vi "Core-ErrorHandler.vi"(7 "Ctrl-Refs":T1, 8 "Err-I":errorcluster, 9 "DaqQ-I":refnum<queue>, 10 "MainQ-I":refnum<queue>, 11 "ErrQ-I":refnum<queue>) -> (0 "Err-O":errorcluster)   [LabVIEW 2020]
doc: "CORE-ERROR HANDLING LOOP."
uses:
  Core-CtrlRefs.ctl
panel:
  # ":: Modularized Parallism Templete ::\n- Error Handling Loop -\nby: Techie <HighTechYoung@yahoo.com>\nhttp://www.Vigo-tech.com\nCopyright (C) 2010, Vigo Technologies All Rights Reserved"
  # "Outputs"
  # "Inputs"
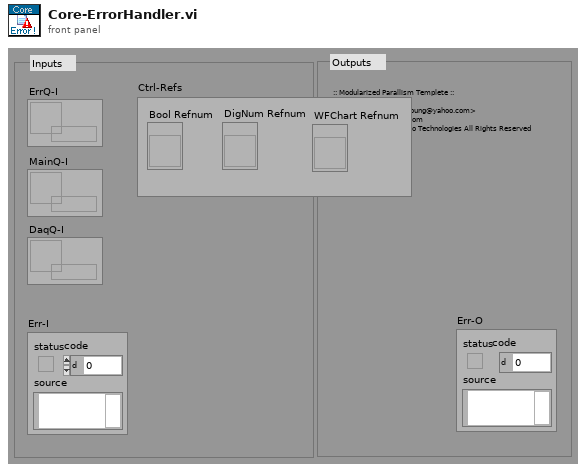
[diagram p1: front panel]
types:
  T1 = typedef "Core-CtrlRefs.ctl" = cluster{"Bool Refnum":refnum<vi>, "DigNum Refnum":refnum<vi>, "WFChart Refnum":refnum<vi>}
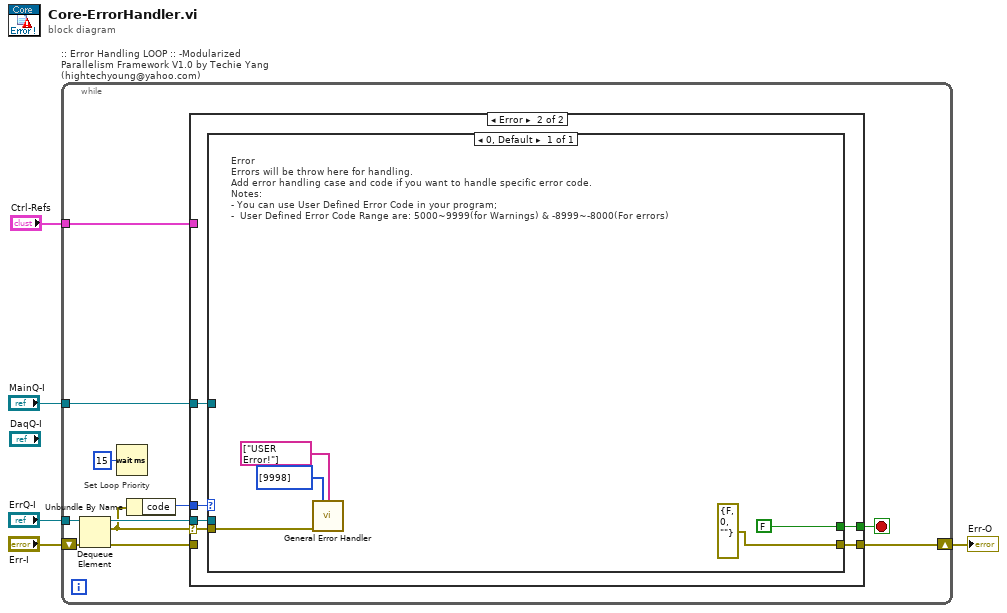
[diagram p0: block diagram]
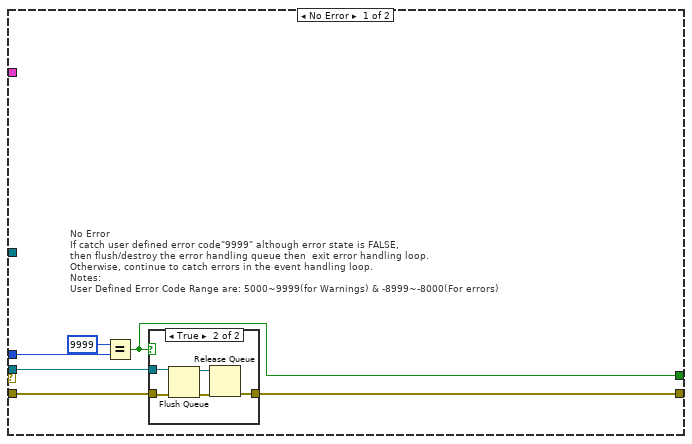
[diagram p2: hidden frame]
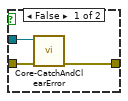
[diagram p3: hidden frame]
diagram:
  n1 = while ":: Error Handling LOOP :: -Modularized Parallelism Framework V1.0 by Techie Yang (hightechyoung@yahoo.com)" {
    tunnel: "ErrQ-I" -> [w16]
    shift-right: [w8] -> w2
    shift-left: "Err-I" -> [w12]
    tunnel: "Ctrl-Refs" -> [w11]
    tunnel: "MainQ-I" -> [w10]
    stop <- w14 stop-if-true
    # "Set Loop Priority"
    n2 = Dequeue Element(queue=w16, error in (no error)=w12) -> (queue out=w13:refnum<queue>, element=w9:errorcluster, error out=w15:errorcluster)  [unwired: 2 out]
    n3 = Wait (ms)(milliseconds to wait=u32 15) -> ()  [unwired: 1 out]
    n4 = Unbundle By Name(w9) -> ("code"=w7:i32)
    n5 = case shown="Error" w9 {
      selector: w9 -> [_ w35]
      tunnel: w15 -> [w22 _]
      tunnel: [w21 w34] -> w8
      tunnel: [w19 w33] -> w14
      tunnel: w13 -> [w20 w31]
      tunnel: w11 -> [_ _]
      tunnel: w10 -> [_ w32]
      tunnel: w7 -> [w18 w36]
      frame No Error {
        # "No Error\nIf catch user defined error code\"9999\" although error state is FALSE, \nthen flush/destroy the error handling queue then  exit error handling loop.\nOtherwise, continue to catch errors in the event handling loop.\nNotes:\nUser Defined Error Code Range are: 5000~9999(for Warnings) & -8999~-8000(For errors)"
        n6 = Equal?(x=9999, y=w18) -> (x = y?=w19:bool)
        n7 = case shown="True" w19 {
          tunnel: w22 -> [w24 w29]
          tunnel: [w23 w28] -> w21
          tunnel: w20 -> [w25 w27]
          frame False {
            n8 = call "Core-CatchAndClearError.vi"("Err-I"=w24, "ErrQ-I"=w25) -> ("Err-O"=w23:errorcluster)  [unwired: 9 in]
          }
          frame True {
            n9 = Flush Queue(queue=w27, error in (no error)=w29) -> (queue out=w30:refnum<queue>, error out=w26:errorcluster)  [unwired: 1 out]
            n10 = Release Queue(queue=w30, error in (no error)=w26) -> (error out=w28:errorcluster)  [unwired: 3 out]
          }
        }
      }
      frame Error {
        n11 = case shown="0, Default" w36 {
          tunnel: w35 -> [w39]
          tunnel: [errorcluster {"status"=FALSE, "code"=0, "source"=""} ("error out")] -> w34
          tunnel: [FALSE] -> w33
          tunnel: w32 -> [_]
          tunnel: w31 -> [_]
          frame 0, Default {
            # "Error\nErrors will be throw here for handling.\nAdd error handling case and code if you want to handle specific error code.\nNotes:\n- You can use User Defined Error Code in your program;\n-  User Defined Error Code Range are: 5000~9999(for Warnings) & -8999~-8000(For errors)"
            n12 = call <vilib>:"General Error Handler.vi"("[user-defined codes]"=i32[] [9998], "[user-defined descriptions]"=string[] ["USER Error!"], "error in (no error)"=w39) -> ()  [unwired: 8 in, 5 out]
          }
        }
      }
    }
  }
  "Err-O" <- w2
